vi "initialize.vi"(8 "error in (no error)":errorcluster, 11 "Qtegra in":refnum<class "Qtegra.lvclass">) -> (0 "error out":errorcluster, 1 "String Output":string, 2 "initialized?":bool, 3 "Qtegra out":refnum<class "Qtegra.lvclass">)   [LabVIEW 2018, in "Qtegra.lvclass"]
doc: "initializes an instrument; this method is going to be replaced by the same method of the child objects"
uses:
  Qtegra.lvclass
  \\Mac\Home/my data/privat/Software/LabView/MSControlSuite_Code/MSControl/Classes/Instrument/instrument.lvclass
  global variables.vi
  instrument.lvclass
  StatusLog/StatusLog.lvclass
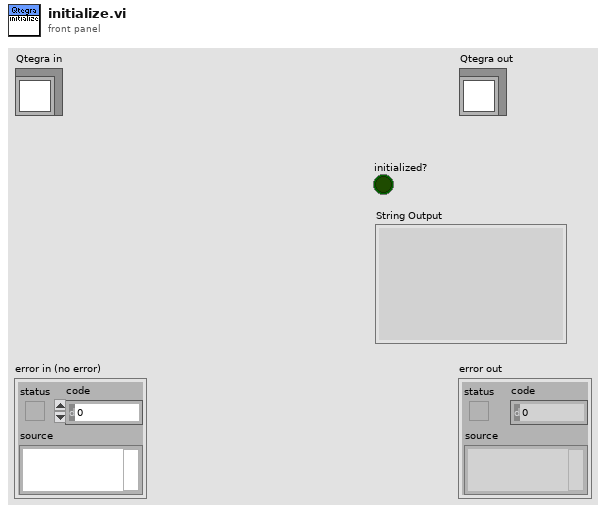
[diagram p1: front panel]
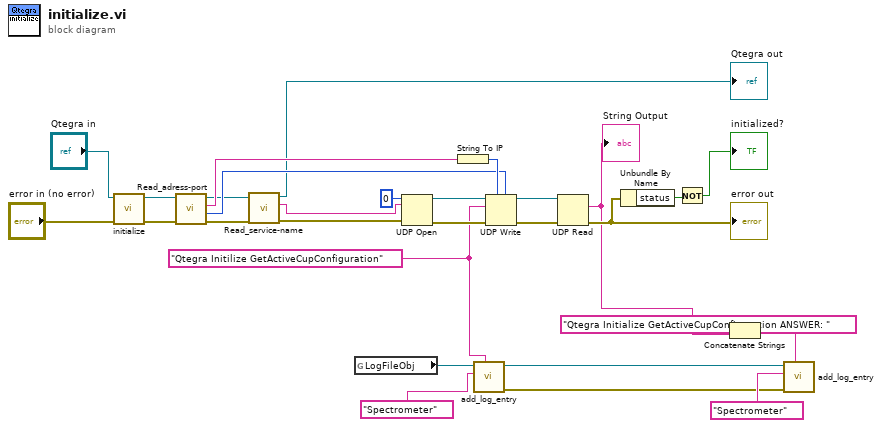
[diagram p0: block diagram]
diagram:
  w2 = "Qtegra Initilize GetActiveCupConfiguration" ("data in")
  n1 = call-parent "initialize.vi"("error in (no error)"="error in (no error)", "instrument in"="Qtegra in") -> ("error out"=w26:errorcluster, "instrument out"=w27:refnum<class "Qtegra.lvclass">)  [unwired: 6 in, 2 out]
  n2 = call "Read_adress-port.vi"("error in (no error)"=w26, "instrument in"=w27) -> ("error out"=w14:errorcluster, "port number"=w15:i32, "adress"=w25:string, "instrument out"=w13:refnum<class "Qtegra.lvclass">)  [unwired: 6 in]
  n3 = call-dynamic "Read_service-name.vi"("error in (no error)"=w14, "instrument in"=w13) -> ("error out"=w11:errorcluster, "service name"=w10:string, "instrument out"=→"Qtegra out":refnum<class "Qtegra.lvclass">)  [unwired: 7 in]
  n4 = global read "global variables.vi" "LogFileObj"() -> (w7:refnum<class "StatusLog.lvclass">)
  n5 = UDP Open(8:w11, 10:w10, 11:u16 0 ("port")) -> (port=w21:refnum<k16>, 0:w22:errorcluster)  [unwired: 2 in, 1 out]
  n6 = String To IP(1:w25) -> (0:w24:u32)
  n7 = call-dynamic "add_log_entry.vi"("new entry"=w2, "log identifiers"="Spectrometer", "StatusLog in"=w7) -> ("error out"=w3:errorcluster, "StatusLog out"=w6:refnum<class "StatusLog.lvclass">)  [unwired: 5 in]
  n8 = UDP Write(address=w24, port or service name=w15, connection ID=w21, data in=w2, 8:w22) -> (error out=w19:errorcluster, 3:w20:refnum<k16>)  [unwired: 1 in]
  n9 = UDP Read(connection ID=w20, 8:w19) -> (data out=w1:string, error out=w18:errorcluster)  [unwired: 2 in, 3 out]
  "error out" <- w18
  "String Output" <- w1
  n10 = Unbundle By Name(w18) -> ("status"=w17:bool)
  n11 = Not(x=w17) -> (.not. x?=→"initialized?":bool)
  n12 = Concatenate Strings("Qtegra Initialize GetActiveCupConfiguration ANSWER: ", w1) -> (w4:string)
  n13 = call-dynamic "add_log_entry.vi"("new entry"=w4, "error in (no error)"=w3, "log identifiers"="Spectrometer", "StatusLog in"=w6) -> ()  [unwired: 4 in, 2 out]
